vi "LabVIEW-MATLAB Timestamp Comparison.vi"() -> ()   [LabVIEW 2020]
uses:
  32e5ddda-8e47-42af-be55-55bcc991336f.vi
  <extravilib>/ChannelInstances/Stream-a[.](dbl)/Read With Abort.vi
  <vilib>/Utility/High Resolution Relative Seconds.vi
  <extravilib>/ChannelInstances/Stream-a[.](dbl)/Write With Abort.vi
  <extravilib>/ChannelInstances/Stream-a[.](dbl)/EndpointRead.vi
  <extravilib>/ChannelInstances/Stream-a[.](dbl)/Endpoint.vi
  <extravilib>/ChannelInstances/Stream-a[.](dbl)/Instantiate.vi
  <extravilib>/ChannelInstances/Stream-a[.](dbl)/)Channel.vi
  <resource>/ChannelSupport/_ChannelSupport/WaitIfNeeded.vi
  <extravilib>/ChannelInstances/Stream-a[.](dbl).lvlib
panel:
  out "XY Graph":cluster{"Y - mean(Y)":dbl[], dbl[]}(graph)
  in  "stop":bool
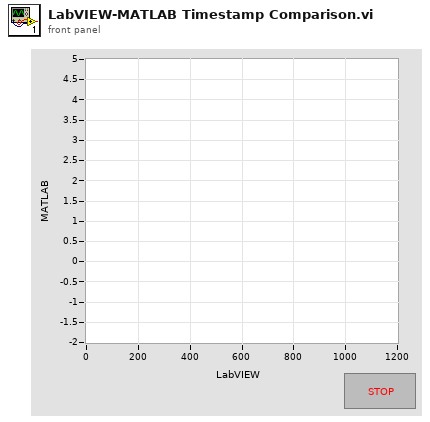
[diagram p1: front panel]
types:
  T1 = typedef "Stream-a[.](dbl).lvlib/)Channel.ctl" = refnum<queue>
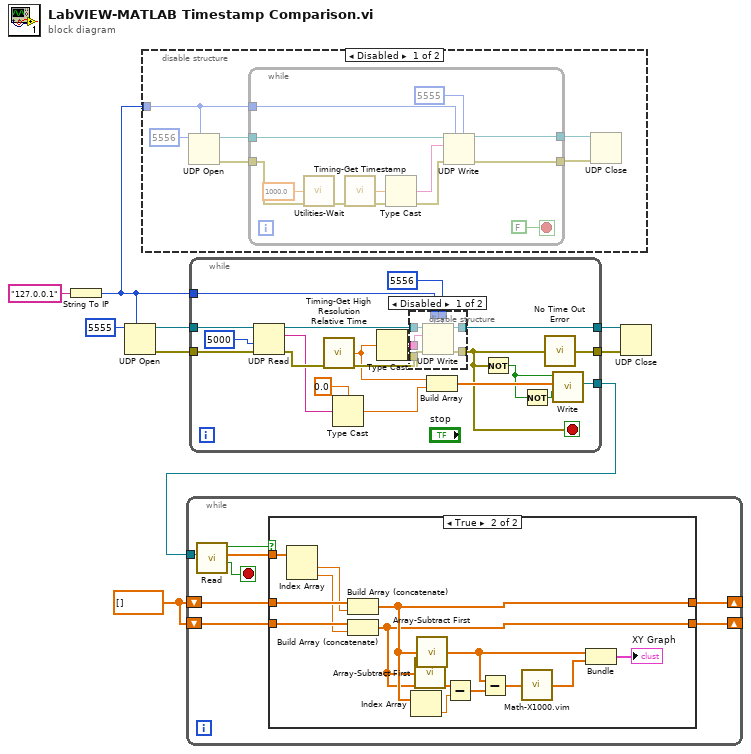
[diagram p0: block diagram]
diagram:
  w3 = dbl[] []
  n1 = String To IP(1:"127.0.0.1" ("name")) -> (0:w1:u32)
  n2 = UDP Open(7:w1, 11:u16 5555 ("port")) -> (port=w8:refnum<k16>, 0:w7:errorcluster)  [unwired: 3 in, 1 out]
  n3 = disable-structure shown="Disabled" {
    disable-tunnel: w1 -> [w12 _]
    frame Disabled {
      n4 = UDP Open(7:w12, 11:u16 5556 ("port")) -> (port=w14:refnum<k16>, 0:w13:errorcluster)  [unwired: 3 in, 1 out]
      n5 = while {
        tunnel: w14 -> [w24]
        tunnel: w13 -> [w27]
        tunnel: w12 -> [w23]
        tunnel: [w18] -> w11
        tunnel: [w17] -> w10
        stop <- FALSE stop-if-true
        n6 = call "Utilities-Wait.vi"("milliseconds to wait"=1000.0, "error in (no error)"=w27) -> ("error out"=w25:errorcluster)  [unwired: 13 in]
        n7 = call "Timing-Get Timestamp.vi"("error in (no error)"=w25) -> ("double precision float"=w20:dbl, "error out"=w21:errorcluster)  [unwired: 13 in]
        n8 = Type Cast(x=w20) -> (*(type *) &x=w19:string)  [unwired: 1 in]
        n9 = UDP Write(address=w23, port or service name=u16 5555 ("port"), connection ID=w24, data in=w19, 8:w21) -> (error out=w18:errorcluster, 3:w17:refnum<k16>)  [unwired: 1 in]
      }
      n10 = UDP Close(connection ID=w10, 8:w11) -> ()  [unwired: 2 out]
    }
    frame Enabled {
    }
  }
  n11 = while {
    tunnel: w8 -> [w47]
    tunnel: w7 -> [w39]
    tunnel: [w37] -> w6
    tunnel: [w40] -> w5
    tunnel: [w42] -> w4
    tunnel: w1 -> [w34]
    stop <- w30 stop-if-true
    n12 = UDP Read(connection ID=w47, timeout ms (25000)=5000, 8:w39) -> (data out=w31:string, error out=w46:errorcluster, 3:w38:refnum<k16>)  [unwired: 1 in, 2 out]
    n13 = call "Timing-Get High Resolution Relative Time.vi"("error in (no error)"=w46) -> ("double precision float"=w35:dbl, "error out"=w36:errorcluster)  [unwired: 13 in]
    n14 = Type Cast(type=0.0, x=w31) -> (*(type *) &x=w44:dbl)
    n15 = Type Cast(x=w35) -> (*(type *) &x=w32:string)  [unwired: 1 in]
    n16 = disable-structure shown="Disabled" {
      disable-tunnel: w38 -> [w54 w56]
      disable-tunnel: [w53 w56] -> w37
      disable-tunnel: w36 -> [w52 w55]
      disable-tunnel: [w51 w55] -> w30
      disable-tunnel: w34 -> [w50 _]
      disable-tunnel: u16 5556 ("port") -> [w49 _]
      disable-tunnel: w32 -> [w48 _]
      frame Disabled {
        n17 = UDP Write(address=w50, port or service name=w49, connection ID=w54, data in=w48, 8:w52) -> (error out=w51:errorcluster, 3:w53:refnum<k16>)  [unwired: 1 in]
      }
      frame Enabled {
      }
    }
    n18 = Build Array(w35, w44) -> (w43:dbl[])
    n19 = Not(x=w30) -> (.not. x?=w29:bool)
    n20 = Not(x=w29) -> (.not. x?=w28:bool)
    n21 = call "No Time Out Error.vi"("error in"=w30) -> ("error out"=w40:errorcluster)  [unwired: 14 in]
    n22 = call <extravilib>:"Write.vi"("last element? (F)"=w28, "element"=w43, "element valid? (T)"=w29) -> ("channel"=w42:T1)  [unwired: 6 in, 2 out]
  }
  n23 = while {
    tunnel: w4 -> [w64]
    shift-right: [w59] -> _
    shift-left: w3 -> [w61]
    shift-right: [w58] -> _
    shift-left: w3 -> [w60]
    stop <- w63 stop-if-true
    n24 = call <extravilib>:"Read.vi"("channel"=w64) -> ("last element?"=w63:bool, "element"=w62:dbl[], "element valid?"=w57:bool)  [unwired: 6 in, 2 out]
    n25 = case shown="True" w57 {
      tunnel: w62 -> [_ w79]
      tunnel: w61 -> [w66 w78]
      tunnel: w60 -> [w65 w76]
      tunnel: [w66 w69] -> w59
      tunnel: [w65 w68] -> w58
      frame False {
      }
      frame True {
        n26 = Index Array(array=w79) -> (element #1=w77:dbl, element #2=w75:dbl)  [unwired: 2 in]
        n27 = Build Array (concatenate)(w78, w77) -> (w69:dbl[])
        n28 = Build Array (concatenate)(w76, w75) -> (w68:dbl[])
        n29 = Index Array(array=w69) -> (element=w70:dbl)  [unwired: 1 in]
        n30 = call "Array-Subtract First.vi"("Y"=w68) -> ()  [unwired: 4 in, 1 out]
        n31 = call "Array-Subtract First.vi"("Y"=w69) -> ("Y - mean(Y)"=w73:dbl[])  [unwired: 4 in]
        n32 = Subtract(x=w68, y=w70) -> (x-y=w67:dbl[])
        n33 = Subtract(x=w73, y=w67) -> (x-y=w74:dbl[])
        n34 = call "Math-X1000.vim"("X"=w74) -> ("1000X"=w71:dbl[])
        n35 = Bundle("Y - mean(Y)"=w73, "1000X"=w71) -> (→"XY Graph":cluster{"Y - mean(Y)":dbl[], "1000X":dbl[]})  [unwired: 1 in]
      }
    }
  }
  n36 = UDP Close(connection ID=w6, 8:w5) -> ()  [unwired: 2 out]
